vi "CAN close.vi"(0 "Channel is active":refnum<vi>, 1 "CAN controller is started":refnum<vi>, 2 "stop":bool, 3 "CAN Control Handle":u32, 4 "Device Handle":u32, 5 "CAN Channel Handle out":u32) -> ()   [LabVIEW 2011]
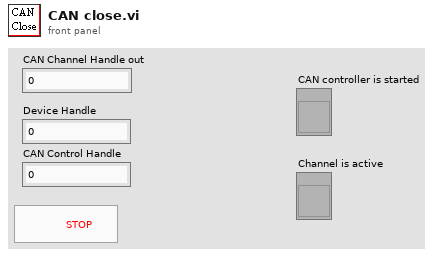
[diagram p1: front panel]
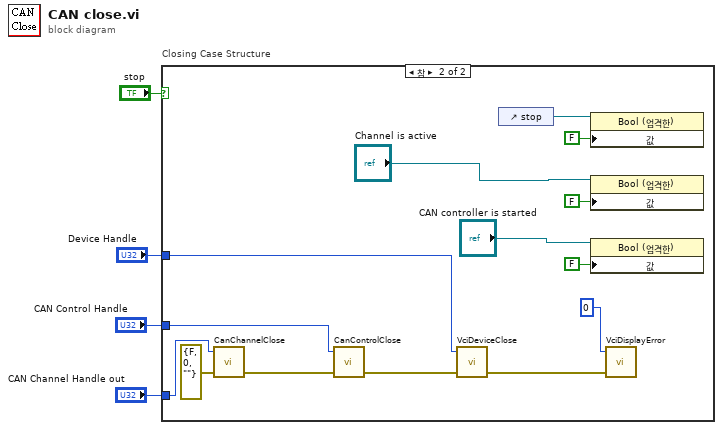
[diagram p0: block diagram]
diagram:
  n1 = case "Closing Case Structure" shown="참" "stop" {
    tunnel: "CAN Channel Handle out" -> [_ w18]
    tunnel: "Device Handle" -> [_ w9]
    tunnel: "CAN Control Handle" -> [_ w17]
    frame False {
    }
    frame True {
      n2 = call "CanChannelClose.vi"("error in"=errorcluster {"status"=FALSE, "code"=0, "source"=""}, "CAN Channel Handle"=w18) -> ("error out"=w12:errorcluster)  [unwired: 3 in]
      n3 = call "CanControlClose.vi"("error in"=w12, "CAN Control Handle"=w17) -> ("error out"=w11:errorcluster)  [unwired: 3 in]
      n4 = call "VciDeviceClose.vi"("error in"=w11, "Device Handle"=w9) -> ("error out"=w10:errorcluster)  [unwired: 3 in]
      n5 = control-ref of="stop"() -> (w13:refnum<vi>)
      n6 = property class="Bool (엄격한)"(reference=w13, "값"=FALSE ("Value")) -> ()  [unwired: 1 in, 2 out]
      n7 = property class="Bool (엄격한)"(reference="Channel is active", "값"=FALSE ("Value")) -> ()  [unwired: 1 in, 2 out]
      n8 = property class="Bool (엄격한)"(reference="CAN controller is started", "값"=FALSE ("Value")) -> ()  [unwired: 1 in, 2 out]
      n9 = call "VciDisplayError.vi"("error in"=w10, "HWND Parent"=u32 0) -> ()  [unwired: 4 in]
    }
  }
